vi "五参数水样测试.vi"(11 "启动参数":T1={"测量模式"=enum."水样测试", "数据标记表"="N", "测量时间"=3.0}) -> ()   [LabVIEW 2016, in "斯坦道仪器.lvlib"]
uses:
  PLC/PLC.lvlib
panel:
  out "枚举":T2(ring)
  out "状态":string
  out "数值":i32
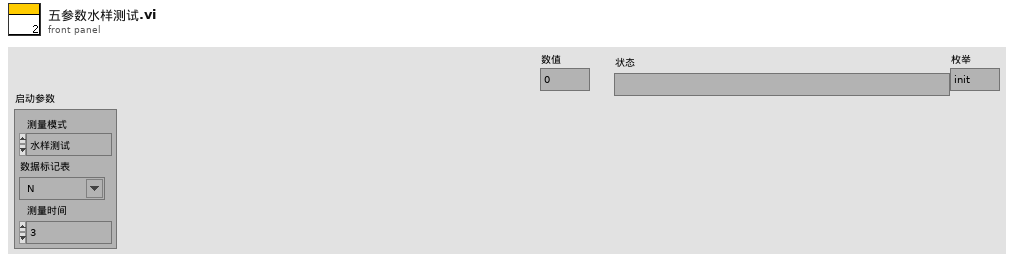
[diagram p1: front panel]
types:
  T1 = cluster{"测量模式":enum16{"待机", "水样测试", "标样核查", "零点核查", "跨度核查", "空白测试", "平行样测试", "加标回收", "空白校准", "标样校准", "初始化（清洗）"}, "数据标记表":string, "测量时间":dbl}
  T2 = enum16{"init", "开机", "启动测量", "读取测量值", "存储数据", "关闭测量", "关机", "结束"}
  T3 = cluster{"时间标识":timestamp, "设备":string, "日志信息":string, "流程参数":string}
  T4 = cluster{"系统时间":timestamp, "工作状态":u16, "测量模式":u16, "告警代码":enum16{"无告警", "缺试剂告警", "缺水样告警", "缺蒸馏水告警", "缺标液告警", "仪表漏液告警", "标定异常告警", "超量程告警", "加热异常", "低试剂预警", "超上限告警", "超下限告警", "仪表内部其他异常", "滴定异常告警", "电极异常告警", "量程切换告警", "参数设置告警", "PH电极电位异常", "电导率电极异常", "浊度光度异常", "溶解氧电极异常", "溶解氧光强异常", "温度异常告警", "PH异常告警", "溶解氧异常告警", "电导率异常告警", "浊度异常告警", "叶绿素异常告警", "藻密度异常告警", "蓝绿藻异常告警", "ORP异常告警", "氨氮异常告警", "清洁刷异常告警", "SD卡异常告警", "蓝牙异常告警", "Wifi异常告警", "流程异常告警"}, "故障代码":enum16{"无故障", "电机故障", "温度故障", "通讯故障", "滴定故障"}, "日志代码":u16, "软件版本":string}
  T5 = enum16{"待机", "水样测试", "标样核查", "零点核查", "跨度核查", "空白测试", "平行样测试", "加标回收", "空白校准", "标样校准", "初始化（清洗）"}
  T6 = cluster{"水温":dbl, "pH":dbl, "DO":dbl, "Cond":dbl, "Turb":dbl, "叶绿素":dbl, "藻密度":dbl, "蓝绿藻":dbl, "ORP":dbl, "NH3N":dbl}
  T7 = cluster{"数据标记表":string, "测量模式":enum16{"待机", "水样测试", "标样核查", "零点核查", "跨度核查", "空白测试", "平行样测试", "加标回收", "空白校准", "标样校准", "初始化（清洗）"}, "database":string}
  T8 = cluster{"因子编码":string, "单位":string, "标样参考值":sgl, "水样数据时间":timestamp, "水样实测值":sgl, "水样数据标识":string, "K":sgl, "B":sgl, "T":sgl, "H":sgl, "水深":sgl, "探头温度":sgl}
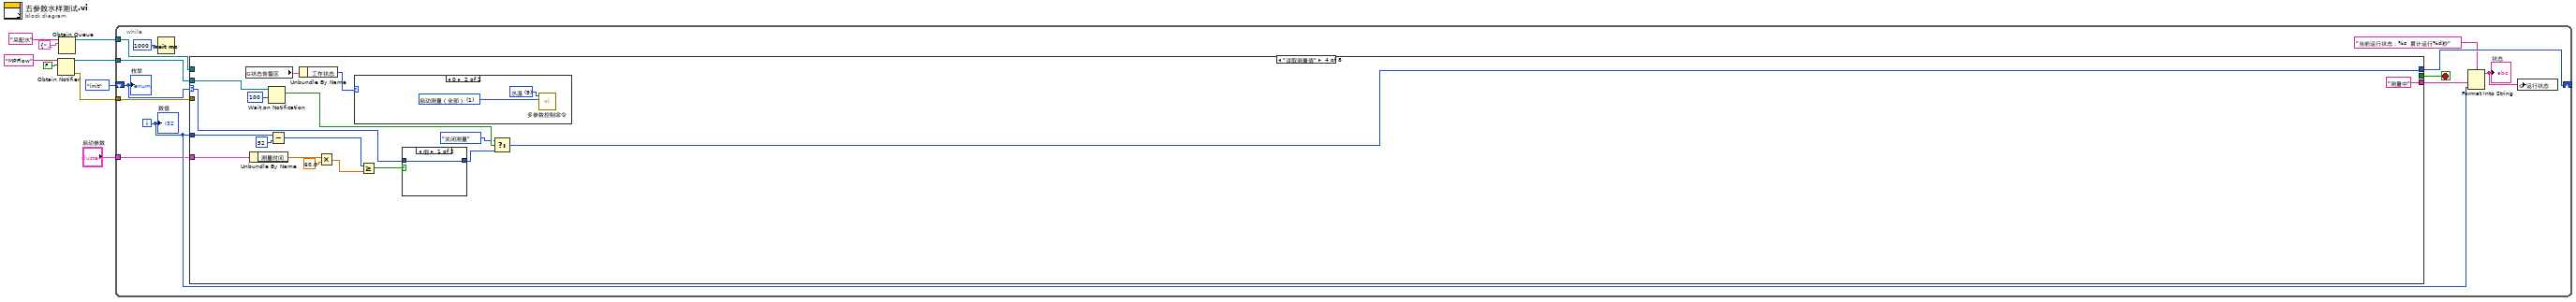
[diagram p0: block diagram]
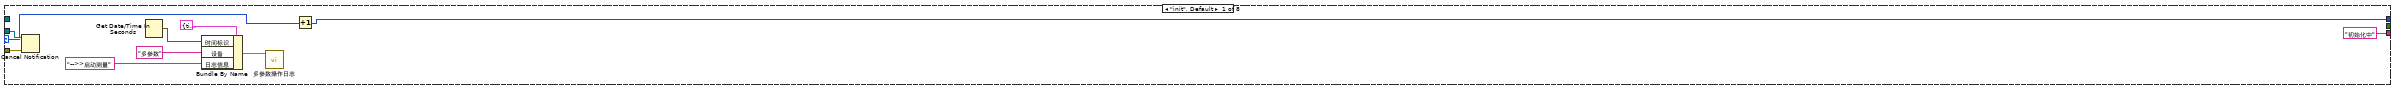
[diagram p2: hidden frame]
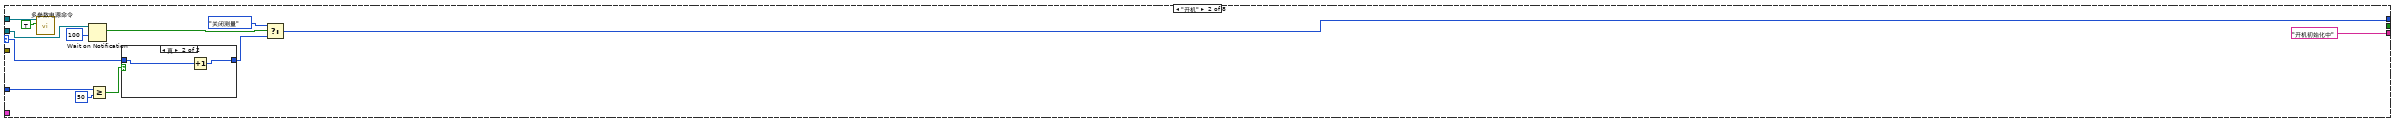
[diagram p3: hidden frame]
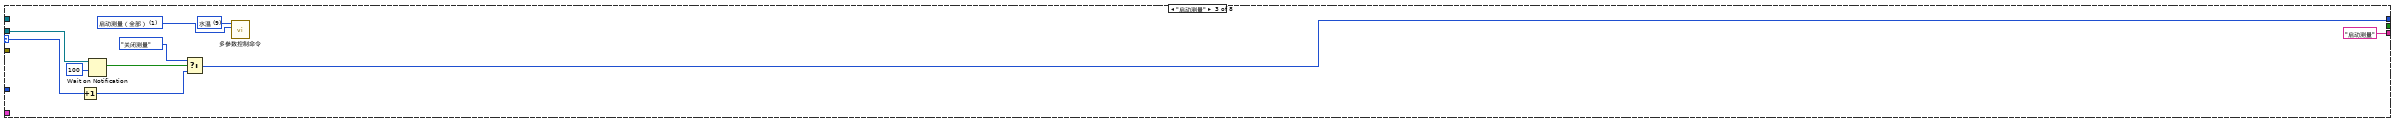
[diagram p5: hidden frame]
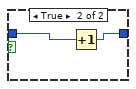
[diagram p7: hidden frame]
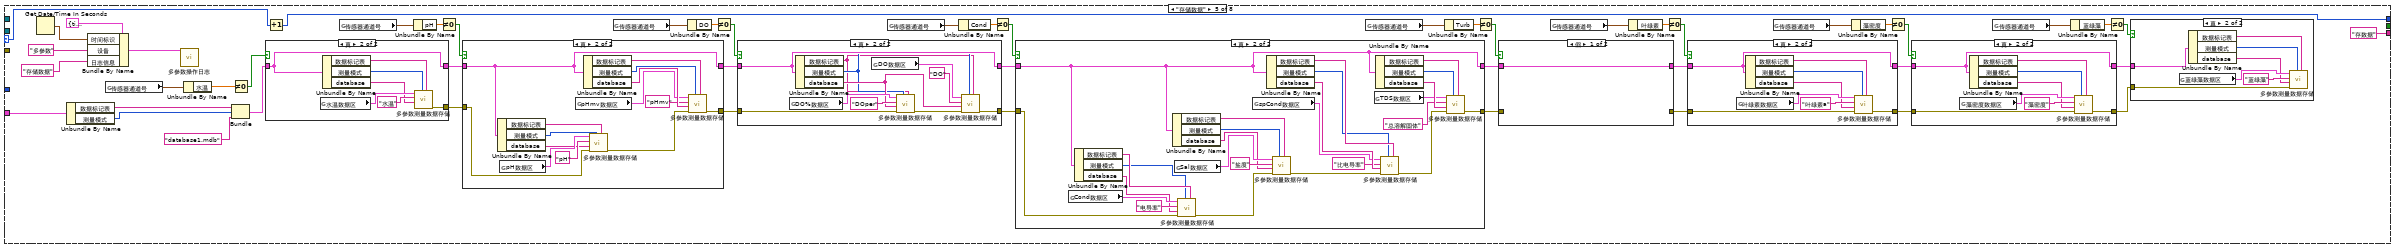
[diagram p8: hidden frame]
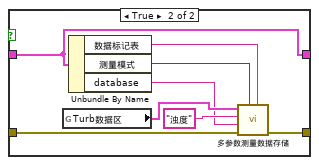
[diagram p12: hidden frame]
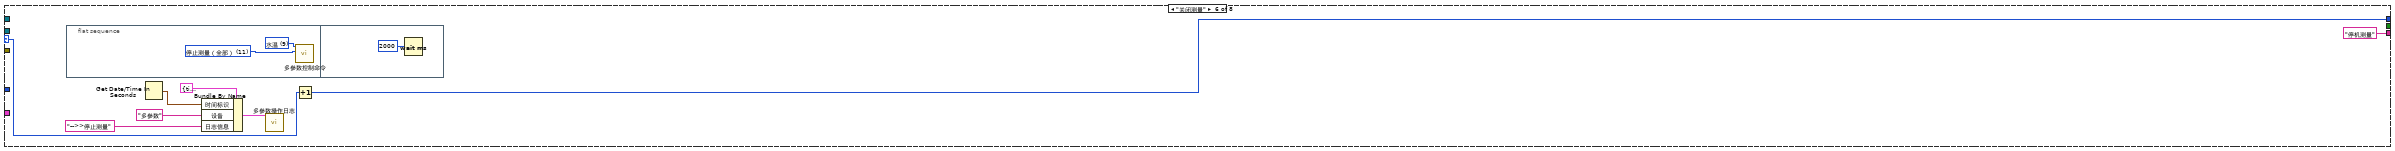
[diagram p17: hidden frame]
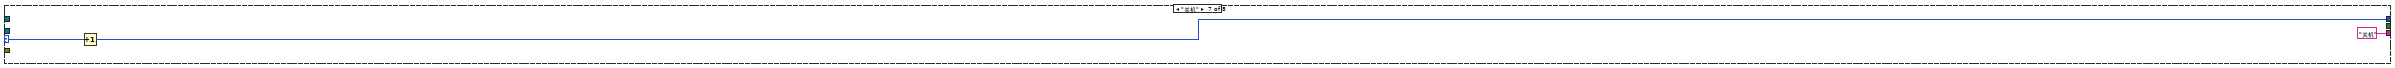
[diagram p18: hidden frame]
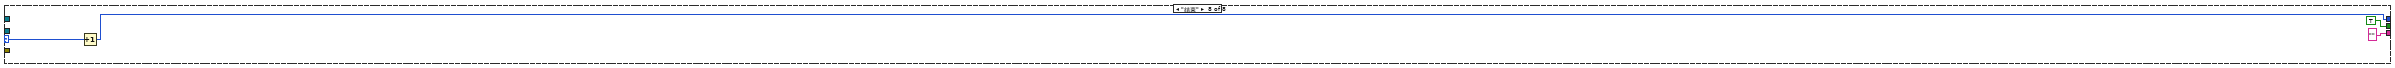
[diagram p19: hidden frame]
diagram:
  n1 = Obtain Notifier(name (unnamed)="MPFlow" ("名称（未命名）"), notification data type=FALSE) -> (notifier out=w6:refnum<notifier>, error out=w5:errorcluster)  [unwired: 2 in, 1 out]
  n2 = Obtain Queue(name (unnamed)="采配水" ("名称（未命名）"), element data type=cluster{"命令":string, "数据":variant} {"命令"="", "数据"=variant}) -> (queue out=w1:refnum<queue>)  [unwired: 3 in, 2 out]
  n3 = while {
    shift-right: [w17] -> _
    shift-left: T2."init" ("枚举") -> [w21]
    tunnel: w6 -> [w19]
    tunnel: w5 -> [w18]
    tunnel: "启动参数" -> [w11]
    tunnel: w1 -> [w10]
    i -> [w13]
    stop <- w20 stop-if-true
    n4 = Wait (ms)(milliseconds to wait=u32 1000 ("等待时间（毫秒）")) -> ()  [unwired: 1 out]
    n5 = case shown="\"读取测量值\"" w21 {
      selector: w21 -> [w29 w44 w57 w75 w131 w235 w241 w244]
      tunnel: [_ _ _ _ _ _ _ TRUE] -> w20
      tunnel: w19 -> [w31 w39 w56 w72 _ _ _ _]
      tunnel: w18 -> [w30 _ _ _ _ _ _ _]
      tunnel: [w28 w37 w53 w70 w130 w234 w240 w243] -> w17
      tunnel: w13 -> [_ w43 _ w62 _ _ _ _]
      tunnel: ["初始化中" ("状态") "开机初始化中" ("状态") "启动测量" ("状态") "测量中" ("状态") "存数据" ("状态") "停机测量" ("状态") "关机" ("状态") "" ("状态")] -> w14
      tunnel: w11 -> [_ _ _ w66 w128 _ _ _]
      tunnel: w10 -> [_ w33 _ _ _ _ _ _]
      frame "init", Default {
        n6 = Cancel Notification(0:w31, 3:w30) -> ()  [unwired: 3 out]
        n7 = Get Date/Time In Seconds() -> (seconds since 1Jan1904=w25:timestamp)
        n8 = Bundle By Name(cluster=T3 {"时间标识"=timestamp(0 s since 1904-01-01), "设备"="", "日志信息"="", "流程参数"=""} ("data in"), "时间标识"=w25, "设备"="多参数", "日志信息"="-->>启动测量") -> (w24:T3)
        n9 = call "多参数操作日志.vi"("data in"=w24) -> ()  [unwired: 10 in, 1 out]
        n10 = Increment(x=w29) -> (x+1=w28:T2)
      }
      frame "开机" {
        n11 = call "多参数电源命令.vi"("通电/断电"=TRUE, "队列"=w33) -> ()  [unwired: 9 in, 1 out]
        n12 = Wait on Notification(notifier=w39, timeout in ms (-1)=100 ("超时毫秒(-1)")) -> (notification=w40:bool)  [unwired: 2 in, 3 out]
        n13 = Greater Or Equal?(x=w43, y=50) -> (x >= y?=w41:bool)
        n14 = case shown="真" w41 {
          tunnel: w44 -> [w45 w47]
          tunnel: [w45 w46] -> w38
          frame False {
          }
          frame True {
            n15 = Increment(x=w47) -> (x+1=w46:T2)
          }
        }
        n16 = Select(t=T2."关闭测量" ("枚举"), s=w40, f=w38) -> (s? t:f=w37:T2)
      }
      frame "启动测量" {
        w48 = u16 1 items=["启动测量（全部）"=1, "初始化（清洗）"=10, "停止测量（全部）"=11, "校时"=13, "启动测量（单个传感器）"=19, "停止测量（单个传感器）"=20] ("控制命令")
        w49 = u16 9 items=["氨氮"=3, "水温"=9, "pH值"=10, "溶解氧"=11, "电导率"=12, "浊度"=13, "叶绿素a"=14, "藻密度"=15, "蓝绿藻"=16, "氧化还原电位"=17, "溶解氧%"=18, "盐度"=19] ("站号")
        n17 = Increment(x=w57) -> (x+1=w54:T2)
        n18 = Wait on Notification(notifier=w56, timeout in ms (-1)=100 ("超时毫秒(-1)")) -> (notification=w55:bool)  [unwired: 2 in, 3 out]
        n19 = Select(t=T2."关闭测量" ("枚举"), s=w55, f=w54) -> (s? t:f=w53:T2)
        n20 = call "多参数控制命令.vi"("控制命令"=w48, "站号"=w49) -> ()  [unwired: 9 in, 1 out]
      }
      frame "读取测量值" {
        n21 = global read "多参数全局变量.vi" "状态告警区"() -> (w59:T4)
        n22 = Unbundle By Name(w66) -> ("测量时间"=w65:dbl)
        n23 = Wait on Notification(notifier=w72, timeout in ms (-1)=100 ("超时毫秒(-1)")) -> (notification=w73:bool)  [unwired: 2 in, 3 out]
        n24 = Subtract(x=w62, y=52) -> (x-y=w61:i32)
        n25 = Unbundle By Name(w59) -> ("工作状态"=w58:u16)
        n26 = Multiply(x=w65, y=60.0) -> (x*y=w63:dbl)
        n27 = case shown="0" w58 {
          frame Default {
          }
          frame 0 {
            w76 = u16 1 items=["启动测量（全部）"=1, "初始化（清洗）"=10, "停止测量（全部）"=11, "校时"=13, "启动测量（单个传感器）"=19, "停止测量（单个传感器）"=20] ("控制命令")
            w77 = u16 9 items=["氨氮"=3, "水温"=9, "pH值"=10, "溶解氧"=11, "电导率"=12, "浊度"=13, "叶绿素a"=14, "藻密度"=15, "蓝绿藻"=16, "氧化还原电位"=17, "溶解氧%"=18, "盐度"=19] ("站号")
            n28 = call "多参数控制命令.vi"("控制命令"=w76, "站号"=w77) -> ()  [unwired: 9 in, 1 out]
          }
        }
        n29 = Greater Or Equal?(x=w61, y=w63) -> (x >= y?=w74:bool)
        n30 = case shown="假" w74 {
          tunnel: w75 -> [w78 w80]
          tunnel: [w78 w79] -> w71
          frame False {
          }
          frame True {
            n31 = Increment(x=w80) -> (x+1=w79:T2)
          }
        }
        n32 = Select(t=T2."关闭测量" ("枚举"), s=w73, f=w71) -> (s? t:f=w70:T2)
      }
      frame "存储数据" {
        n33 = Get Date/Time In Seconds() -> (seconds since 1Jan1904=w99:timestamp)
        n34 = Unbundle By Name(w128) -> ("数据标记表"=w107:string, "测量模式"=w106:T5)
        n35 = Bundle By Name(cluster=T3 {"时间标识"=timestamp(0 s since 1904-01-01), "设备"="", "日志信息"="", "流程参数"=""} ("data in"), "时间标识"=w99, "设备"="多参数", "日志信息"="存储数据") -> (w98:T3)
        n36 = global read "多参数全局变量.vi" "传感器通道号"() -> (w123:T6)
        n37 = call "多参数操作日志.vi"("data in"=w98) -> ()  [unwired: 10 in, 1 out]
        n38 = Unbundle By Name(w123) -> ("水温"=w122:dbl)
        n39 = Not Equal To 0?(x=w122) -> (x != 0?=w121:bool)
        n40 = Bundle("数据标记表"=w107, "测量模式"=w106, "database"="database1.mdb") -> (w105:T7)  [unwired: 1 in]
        n41 = case shown="真" w121 {
          tunnel: [_ w225] -> w127
          tunnel: w105 -> [w220 w224]
          tunnel: [w220 w224] -> w104
          frame False {
          }
          frame True {
            n42 = global read "多参数全局变量.vi" "水温数据区"() -> (w227:T8)
            n43 = Unbundle By Name(w224) -> ("数据标记表"=w223:string, "测量模式"=w222:T5, "database"=w221:string)
            n44 = call "多参数测量数据存储.vi"("数据标记表"=w223, "测量模式"=w222, "database"=w221, "table输入"="水温", "data in"=w227) -> ("error out"=w225:errorcluster)  [unwired: 6 in]
          }
        }
        n45 = Increment(x=w131) -> (x+1=w130:T2)
        n46 = global read "多参数全局变量.vi" "传感器通道号"() -> (w116:T6)
        n47 = Unbundle By Name(w116) -> ("pH"=w115:dbl)
        n48 = Not Equal To 0?(x=w115) -> (x != 0?=w120:bool)
        n49 = case shown="真" w120 {
          tunnel: w127 -> [_ w219]
          tunnel: [_ w208] -> w126
          tunnel: w104 -> [w205 w213]
          tunnel: [w205 w213] -> w102
          frame False {
          }
          frame True {
            n50 = Unbundle By Name(w213) -> ("数据标记表"=w216:string, "测量模式"=w215:T5, "database"=w214:string)
            n51 = global read "多参数全局变量.vi" "pH数据区"() -> (w218:T8)
            n52 = global read "多参数全局变量.vi" "pHmv数据区"() -> (w207:T8)
            n53 = Unbundle By Name(w213) -> ("数据标记表"=w212:string, "测量模式"=w211:T5, "database"=w210:string)
            n54 = call "多参数测量数据存储.vi"("数据标记表"=w216, "测量模式"=w215, "error in (no error)"=w219, "database"=w214, "table输入"="pH", "data in"=w218) -> ("error out"=w209:errorcluster)  [unwired: 5 in]
            n55 = call "多参数测量数据存储.vi"("数据标记表"=w212, "测量模式"=w211, "error in (no error)"=w209, "database"=w210, "table输入"="pHmv", "data in"=w207) -> ("error out"=w208:errorcluster)  [unwired: 5 in]
          }
        }
        n56 = global read "多参数全局变量.vi" "传感器通道号"() -> (w114:T6)
        n57 = Unbundle By Name(w114) -> ("DO"=w113:dbl)
        n58 = Not Equal To 0?(x=w113) -> (x != 0?=w119:bool)
        n59 = case shown="真" w119 {
          tunnel: w126 -> [_ w204]
          tunnel: [_ w200] -> w125
          tunnel: [w193 w197] -> w103
          tunnel: w102 -> [w193 w197]
          frame False {
          }
          frame True {
            n60 = global read "多参数全局变量.vi" "DO%数据区"() -> (w199:T8)
            n61 = Unbundle By Name(w197) -> ("数据标记表"=w194:string, "测量模式"=w195:T5, "database"=w196:string)
            n62 = global read "多参数全局变量.vi" "DO数据区"() -> (w201:T8)
            n63 = call "多参数测量数据存储.vi"("数据标记表"=w194, "测量模式"=w195, "error in (no error)"=w204, "database"=w196, "table输入"="DOper", "data in"=w199) -> ("error out"=w203:errorcluster)  [unwired: 5 in]
            n64 = call "多参数测量数据存储.vi"("数据标记表"=w194, "测量模式"=w195, "error in (no error)"=w203, "database"=w196, "table输入"="DO", "data in"=w201) -> ("error out"=w200:errorcluster)  [unwired: 5 in]
          }
        }
        n65 = global read "多参数全局变量.vi" "传感器通道号"() -> (w112:T6)
        n66 = Unbundle By Name(w112) -> ("Cond"=w111:dbl)
        n67 = Not Equal To 0?(x=w111) -> (x != 0?=w118:bool)
        n68 = case shown="真" w118 {
          tunnel: w125 -> [_ w190]
          tunnel: [_ w171] -> w124
          tunnel: w103 -> [w166 w180]
          tunnel: [w166 w180] -> w101
          frame False {
          }
          frame True {
            n69 = global read "多参数全局变量.vi" "Cond数据区"() -> (w192:T8)
            n70 = Unbundle By Name(w180) -> ("数据标记表"=w185:string, "测量模式"=w184:T5, "database"=w186:string)
            n71 = Unbundle By Name(w180) -> ("数据标记表"=w183:string, "测量模式"=w182:T5, "database"=w181:string)
            n72 = global read "多参数全局变量.vi" "Sal数据区"() -> (w188:T8)
            n73 = call "多参数测量数据存储.vi"("数据标记表"=w185, "测量模式"=w184, "error in (no error)"=w190, "database"=w186, "table输入"="电导率", "data in"=w192) -> ("error out"=w189:errorcluster)  [unwired: 5 in]
            n74 = global read "多参数全局变量.vi" "spCond数据区"() -> (w170:T8)
            n75 = Unbundle By Name(w180) -> ("数据标记表"=w179:string, "测量模式"=w178:T5, "database"=w177:string)
            n76 = call "多参数测量数据存储.vi"("数据标记表"=w183, "测量模式"=w182, "error in (no error)"=w189, "database"=w181, "table输入"="盐度", "data in"=w188) -> ("error out"=w176:errorcluster)  [unwired: 5 in]
            n77 = global read "多参数全局变量.vi" "TDS数据区"() -> (w169:T8)
            n78 = Unbundle By Name(w180) -> ("数据标记表"=w172:string, "测量模式"=w173:T5, "database"=w174:string)
            n79 = call "多参数测量数据存储.vi"("数据标记表"=w179, "测量模式"=w178, "error in (no error)"=w176, "database"=w177, "table输入"="比电导率", "data in"=w170) -> ("error out"=w175:errorcluster)  [unwired: 5 in]
            n80 = call "多参数测量数据存储.vi"("数据标记表"=w172, "测量模式"=w173, "error in (no error)"=w175, "database"=w174, "table输入"="总溶解固体", "data in"=w169) -> ("error out"=w171:errorcluster)  [unwired: 5 in]
          }
        }
        n81 = global read "多参数全局变量.vi" "传感器通道号"() -> (w110:T6)
        n82 = Unbundle By Name(w110) -> ("Turb"=w109:dbl)
        n83 = Not Equal To 0?(x=w109) -> (x != 0?=w117:bool)
        n84 = case shown="假" w117 {
          tunnel: w124 -> [_ w165]
          tunnel: w101 -> [w157 w158]
          tunnel: [_ w159] -> w92
          tunnel: [w157 w158] -> w91
          frame False {
          }
          frame True {
            n85 = global read "多参数全局变量.vi" "Turb数据区"() -> (w164:T8)
            n86 = Unbundle By Name(w158) -> ("数据标记表"=w160:string, "测量模式"=w161:T5, "database"=w162:string)
            n87 = call "多参数测量数据存储.vi"("数据标记表"=w160, "测量模式"=w161, "error in (no error)"=w165, "database"=w162, "table输入"="浊度", "data in"=w164) -> ("error out"=w159:errorcluster)  [unwired: 5 in]
          }
        }
        n88 = global read "多参数全局变量.vi" "传感器通道号"() -> (w94:T6)
        n89 = Unbundle By Name(w94) -> ("叶绿素"=w95:dbl)
        n90 = Not Equal To 0?(x=w95) -> (x != 0?=w93:bool)
        n91 = case shown="真" w93 {
          tunnel: w92 -> [_ w156]
          tunnel: w91 -> [w148 w149]
          tunnel: [_ w150] -> w87
          tunnel: [w148 w149] -> w86
          frame False {
          }
          frame True {
            n92 = global read "多参数全局变量.vi" "叶绿素数据区"() -> (w155:T8)
            n93 = Unbundle By Name(w149) -> ("数据标记表"=w151:string, "测量模式"=w152:T5, "database"=w153:string)
            n94 = call "多参数测量数据存储.vi"("数据标记表"=w151, "测量模式"=w152, "error in (no error)"=w156, "database"=w153, "table输入"="叶绿素a", "data in"=w155) -> ("error out"=w150:errorcluster)  [unwired: 5 in]
          }
        }
        n95 = global read "多参数全局变量.vi" "传感器通道号"() -> (w89:T6)
        n96 = Unbundle By Name(w89) -> ("藻密度"=w88:dbl)
        n97 = Not Equal To 0?(x=w88) -> (x != 0?=w90:bool)
        n98 = case shown="真" w90 {
          tunnel: w87 -> [_ w147]
          tunnel: w86 -> [w139 w141]
          tunnel: [w139 w141] -> w82
          tunnel: [_ w140] -> w81
          frame False {
          }
          frame True {
            n99 = global read "多参数全局变量.vi" "藻密度数据区"() -> (w146:T8)
            n100 = Unbundle By Name(w141) -> ("数据标记表"=w142:string, "测量模式"=w143:T5, "database"=w144:string)
            n101 = call "多参数测量数据存储.vi"("数据标记表"=w142, "测量模式"=w143, "error in (no error)"=w147, "database"=w144, "table输入"="藻密度", "data in"=w146) -> ("error out"=w140:errorcluster)  [unwired: 5 in]
          }
        }
        n102 = global read "多参数全局变量.vi" "传感器通道号"() -> (w84:T6)
        n103 = Unbundle By Name(w84) -> ("蓝绿藻"=w85:dbl)
        n104 = Not Equal To 0?(x=w85) -> (x != 0?=w83:bool)
        n105 = case shown="真" w83 {
          tunnel: w81 -> [_ w138]
          tunnel: w82 -> [_ w135]
          frame False {
          }
          frame True {
            n106 = global read "多参数全局变量.vi" "蓝绿藻数据区"() -> (w137:T8)
            n107 = Unbundle By Name(w135) -> ("数据标记表"=w132:string, "测量模式"=w133:T5, "database"=w134:string)
            n108 = call "多参数测量数据存储.vi"("数据标记表"=w132, "测量模式"=w133, "error in (no error)"=w138, "database"=w134, "table输入"="蓝绿藻", "data in"=w137) -> ()  [unwired: 5 in, 1 out]
          }
        }
      }
      frame "关闭测量" {
        n109 = flat-sequence {
          frame #0 {
            w236 = u16 11 items=["启动测量（全部）"=1, "初始化（清洗）"=10, "停止测量（全部）"=11, "校时"=13, "启动测量（单个传感器）"=19, "停止测量（单个传感器）"=20] ("控制命令")
            w237 = u16 9 items=["氨氮"=3, "水温"=9, "pH值"=10, "溶解氧"=11, "电导率"=12, "浊度"=13, "叶绿素a"=14, "藻密度"=15, "蓝绿藻"=16, "氧化还原电位"=17, "溶解氧%"=18, "盐度"=19] ("站号")
            n110 = call "多参数控制命令.vi"("控制命令"=w236, "站号"=w237) -> ()  [unwired: 9 in, 1 out]
          }
          frame #1 {
            n111 = Wait (ms)(milliseconds to wait=u32 2000 ("等待时间（毫秒）")) -> ()  [unwired: 1 out]
          }
        }
        n112 = Get Date/Time In Seconds() -> (seconds since 1Jan1904=w231:timestamp)
        n113 = Bundle By Name(cluster=T3 {"时间标识"=timestamp(0 s since 1904-01-01), "设备"="", "日志信息"="", "流程参数"=""} ("data in"), "时间标识"=w231, "设备"="多参数", "日志信息"="-->>停止测量") -> (w230:T3)
        n114 = call "多参数操作日志.vi"("data in"=w230) -> ()  [unwired: 10 in, 1 out]
        n115 = Increment(x=w235) -> (x+1=w234:T2)
      }
      frame "关机" {
        n116 = Increment(x=w241) -> (x+1=w240:T2)
      }
      frame "结束" {
        n117 = Increment(x=w244) -> (x+1=w243:T2)
      }
    }
    n118 = Format Into String(format string="当前运行状态：%s  累计运行%d秒" ("格式字符串"), w14, w13) -> (resulting string=w12:string)  [unwired: 2 in, 1 out]
    "状态" <- w12
    n119 = global write "多参数全局变量.vi" "运行状态"(w12) -> ()
    "数值" <- w13
    "枚举" <- w21
  }
